vi "setConnected.vi"(8 "error in (no error)":errorcluster, 10 "connected":bool, 11 "Connection in":refnum<class "Connection.lvclass">) -> (0 "error out":errorcluster, 3 "Connection out":refnum<class "Connection.lvclass">)   [LabVIEW 2013, in "MQTT_Connection.lvlib" / "Connection.lvclass"]
uses:
  Connection.lvclass
  Connection.lvclass/Connection.ctl
  <vilib>/Utility/error.llb/Error Cluster From Error Code.vi
  <vilib>/ErrorRing/Error Ring.xnode
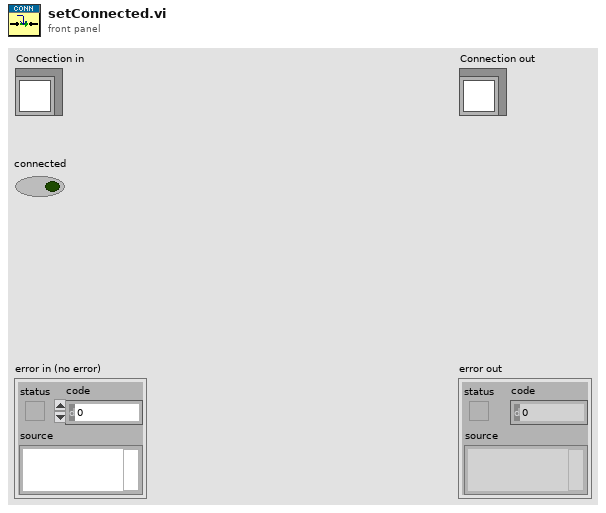
[diagram p1: front panel]
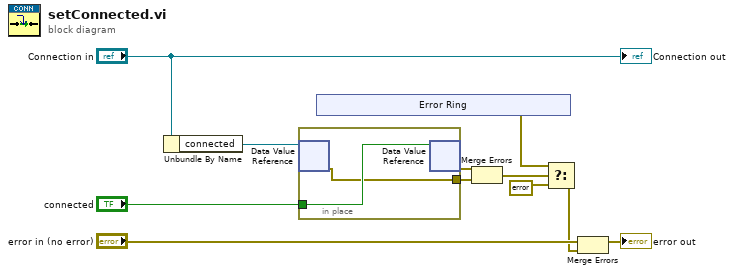
[diagram p0: block diagram]
diagram:
  n1 = Unbundle By Name("Connection in") -> ("connected"=w11:refnum<data-value>)
  n2 = in-place {
    in-place-border: "connected" -> [w13]
    in-place-border: [w12] -> w3
    n3 = in-place-dvr #1(w11) -> (w12:errorcluster)  [unwired: 1 out]
    n4 = in-place-dvr #1(w13) -> (w2:errorcluster)  [unwired: 1 out]
  }
  n5 = xnode "Error Ring"() -> ("error out"=w4:errorcluster)
  n6 = Merge Errors(w2, w3) -> (w6:errorcluster)
  n7 = Select(t=w4, s=w6, f=errorcluster {"status"=FALSE, "code"=0, "source"=""} ("error out")) -> (s? t:f=w1:errorcluster)
  n8 = Merge Errors("error in (no error)", w1) -> (→"error out":errorcluster)
  "Connection out" <- "Connection in"
